vi "Construct RT Seq and Insert Log Trigger.vi"(8 "Error In":errorcluster, 10 "Log Trigger Name (Aliases/CSVSeqLogTrigger)":string="Aliases/CSVSeqLogTrigger", 11 "CSV File":path) -> (0 "Error Out":errorcluster, 3 "RT Seq Ref Out":refnum<k24>)   [LabVIEW 2011]
uses:
  NationalInstruments.VeriStand.RealTimeSequenceDefinitionApi
  NationalInstruments.VeriStand.DataTypes
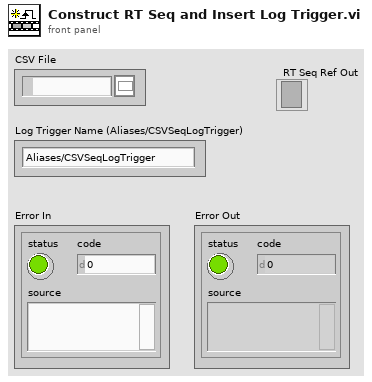
[diagram p1: front panel]
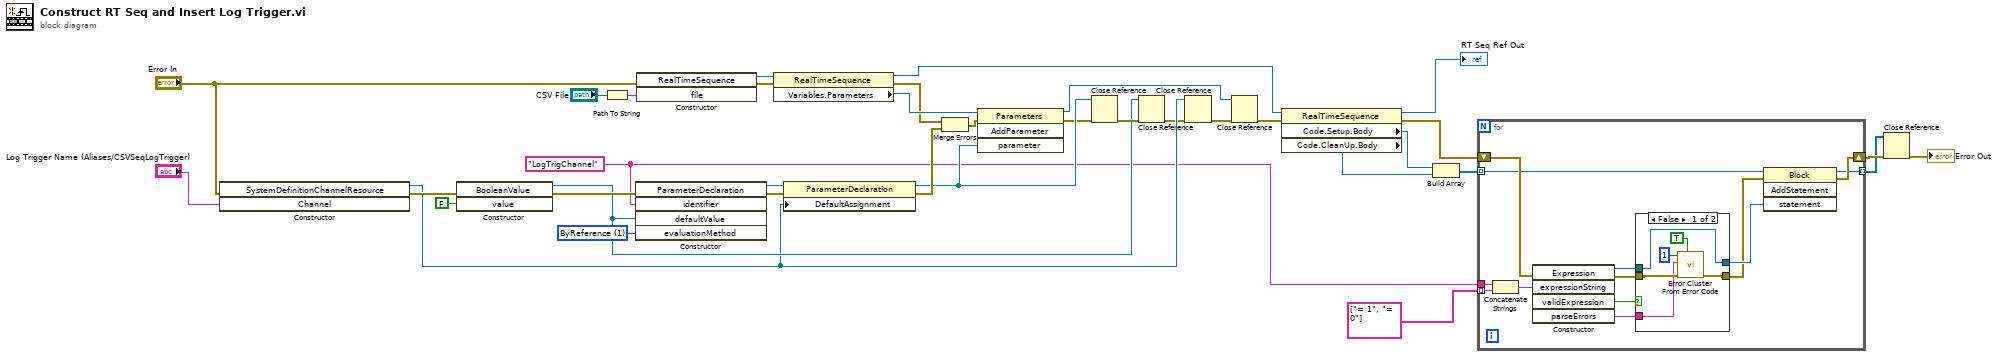
[diagram p0: block diagram]
diagram:
  w31 = 1 items=["ByValue", "ByReference"] ("evaluationMethod")
  w13 = "LogTrigChannel" ("identifier")
  n1 = constructor class="SystemDefinitionChannelResource"(error in="Error In", "Channel"="Log Trigger Name (Aliases/CSVSeqLogTrigger)") -> (reference out=w19:refnum<k24>, error out=w27:errorcluster)  [unwired: 2 in, 2 out]
  n2 = constructor class="BooleanValue"(error in=w27, "value"=FALSE) -> (reference out=w20:refnum<k24>, error out=w33:errorcluster)  [unwired: 2 in, 2 out]
  n3 = Path To String(path="CSV File") -> (string=w35:string)
  n4 = constructor class="ParameterDeclaration"(error in=w33, "identifier"=w13, "defaultValue"=w20, "evaluationMethod"=w31) -> (reference out=w28:refnum<k24>, error out=w29:errorcluster)  [unwired: 2 in, 4 out]
  n5 = constructor class="RealTimeSequence"(error in="Error In", "file"=w35) -> (reference out=w32:refnum<k24>, error out=w34:errorcluster)  [unwired: 2 in, 2 out]
  n6 = property class="RealTimeSequence"(reference=w32, error in=w34) -> (reference out=w14:refnum<k24>, error out=w1:errorcluster, "Variables.Parameters"=w3:refnum<k24>)
  n7 = property class="ParameterDeclaration"(reference=w28, error in=w29, "DefaultAssignment"=w19) -> (reference out=w22:refnum<k24>, error out=w24:errorcluster)
  n8 = Merge Errors(w1, w24) -> (w23:errorcluster)
  n9 = invoke class="Parameters" method="AddParameter"(reference=w3, error in=w23, "parameter"=w22) -> (reference out=w15:refnum<k24>, error out=w17:errorcluster)  [unwired: 1 in, 2 out]
  n10 = Close Reference(reference=w22, error in (no error)=w17) -> (error out=w21:errorcluster)
  n11 = Close Reference(reference=w20, error in (no error)=w21) -> (error out=w18:errorcluster)
  n12 = Close Reference(reference=w19, error in (no error)=w18) -> (error out=w16:errorcluster)
  n13 = Close Reference(reference=w15, error in (no error)=w16) -> (error out=w2:errorcluster)
  n14 = property class="RealTimeSequence"(reference=w14, error in=w2) -> (reference out=→"RT Seq Ref Out":refnum<k24>, error out=w6:errorcluster, "Code.Setup.Body"=w5:refnum<k24>, "Code.CleanUp.Body"=w4:refnum<k24>)
  n15 = Build Array(w5, w4) -> (w12:refnum<k24>[])
  n16 = for {
    tunnel: w13 -> [w49]
    tunnel: w12 -> [w41] mode=indexing
    shift-right: [w38] -> w10
    shift-left: w6 -> [w42]
    tunnel: string[] ["= 1", "= 0"] -> [w39] mode=indexing
    tunnel: [w37] -> w9 mode=indexing
    n17 = Concatenate Strings(w49, w39) -> (w48:string)
    n18 = constructor class="Expression"(error in=w42, "expressionString"=w48) -> (reference out=w43:refnum<k24>, error out=w46:errorcluster, "validExpression"=w47:bool, "parseErrors"=w45:string)  [unwired: 4 in, 2 out]
    n19 = case shown="False" w47 {
      tunnel: [w54 w57] -> w40
      tunnel: w46 -> [w55 w57]
      tunnel: w45 -> [w52 _]
      tunnel: [w51 w56] -> w44
      tunnel: w43 -> [w51 w56]
      frame False {
        n20 = call <vilib>:"Error Cluster From Error Code.vi"("show call chain? (False)"=TRUE, "error in (no error)"=w55, "error message (\"\")"=w52, "error code (0)"=1) -> ("error out"=w54:errorcluster)  [unwired: 5 in]
      }
      frame True {
      }
    }
    n21 = invoke class="Block" method="AddStatement"(reference=w41, error in=w40, "statement"=w44) -> (reference out=w37:refnum<k24>, error out=w38:errorcluster)  [unwired: 1 in, 2 out]
  }
  n22 = Close Reference(reference=w9, error in (no error)=w10) -> (error out=→"Error Out":errorcluster)
